vi "Board Type Enum to Board Design.vi"(11 "which board":T1) -> (3 "Board Design":refnum<class "Board Design.lvclass">)   [LabVIEW 2018, in "Board Design.lvclass"]
uses:
  Board Design.lvclass
  Common/Board Type Enum.ctl
  Basic DAQ Design_class/Basic DAQ Design.lvclass
  C:/GitClones/LGP5-Resources/LVOOP/Board Testing - From Task-Oriented to Object-Oriented/Classes/Board Design_class/Board Design.lvclass
  Elite DAQ Design_class/Elite DAQ Design.lvclass
  GPIB Board Design_class/GPIB Board Design.lvclass
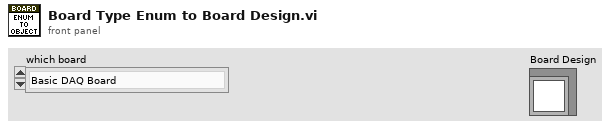
[diagram p1: front panel]
types:
  T1 = typedef "Board Type Enum.ctl" = enum16{"Basic DAQ Board", "Elite DAQ Board", "GPIB Board"}
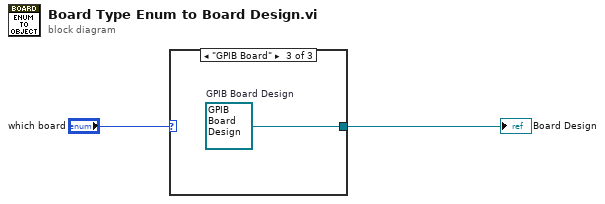
[diagram p0: block diagram]
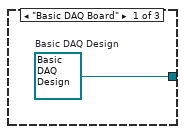
[diagram p2: hidden frame]
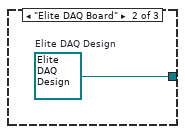
[diagram p3: hidden frame]
diagram:
  n1 = case shown="\"GPIB Board\"" "which board" {
    tunnel: [w3 w4 w5] -> w1
    frame "Basic DAQ Board" {
      w3 = refnum<class "Basic DAQ Design.lvclass"> refnum  # Basic DAQ Design
    }
    frame "Elite DAQ Board" {
      w4 = refnum<class "Elite DAQ Design.lvclass"> refnum  # Elite DAQ Design
    }
    frame "GPIB Board" {
      w5 = refnum<class "GPIB Board Design.lvclass"> refnum  # GPIB Board Design
    }
  }
  "Board Design" <- w1
